vi "NetworkStreamReceiverTemplate.vi"() -> ()   [LabVIEW 2014]
doc: "Use this template to build a producer/consumer design pattern. Use this template when you need to execute a process, such as data analysis, when a data source, such as a triggered acquisition, produces data at an uneven rate and you need to execute the process when the data becomes available."
uses:
  NetworkStreamReceiverState.ctl
  NetworkStreamStateMachineVariable.ctl
  NetworkStreamData.ctl
  NetworkStreamReceiverMainQueueCluster.ctl
  NetworkStreamReceiverStatusEventCluster.ctl
  <vilib>/dex/Stream Element Allocation Mode.ctl
  NetworkStream.lvlib
panel:
  out "Random Session Hash":u64
  out "Network Stream State Indicator":T1
  in  "stop":bool
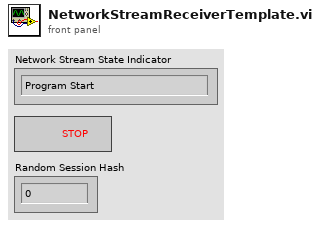
[diagram p1: front panel]
types:
  T1 = typedef "NetworkStream.lvlib/NetworkStreamReceiverState.ctl" = enum16{"Program Start", "Waiting for connection", "Connected", "Connection lost", "Exit", "Unhandled Exception"}
  T2 = typedef "NetworkStream.lvlib/NetworkStreamReceiverStatusEventCluster.ctl" = cluster{"Status":string, "Data":variant, "SequenceNumber":u64}
  T3 = typedef "NetworkStream.lvlib/NetworkStreamReceiverMainQueueCluster.ctl" = cluster{"Command":string, "Data":variant, "SequenceNumber":u64}
  T4 = typedef "NetworkStream.lvlib/NetworkStreamStateMachineVariable.ctl" = cluster{"Network Stream Reader Endpoint":refnum<k21>, "Last Received Sequence Number":u64}
  T5 = typedef "NetworkStream.lvlib/NetworkStreamData.ctl" = cluster{"Command/Status":string, "Data":variant, "Session Hash":u64, "Sequence Number":u64}
  T6 = typedef "Stream Element Allocation Mode.ctl" = u32
  T7 = cluster{"Command/Status":string, "Data":variant, "Sequence Number":u64}
  T8 = cluster{"Status":string, "Data":variant, "Random Session Hash":u64, "SequenceNumberOfFinishedCommand":u64}
  T9 = cluster{"Command":string, "Data":variant, "SequenceNumberOfCommand":u64}
  T10 = cluster{string, "Variant":variant, "SequenceNumber":u64}
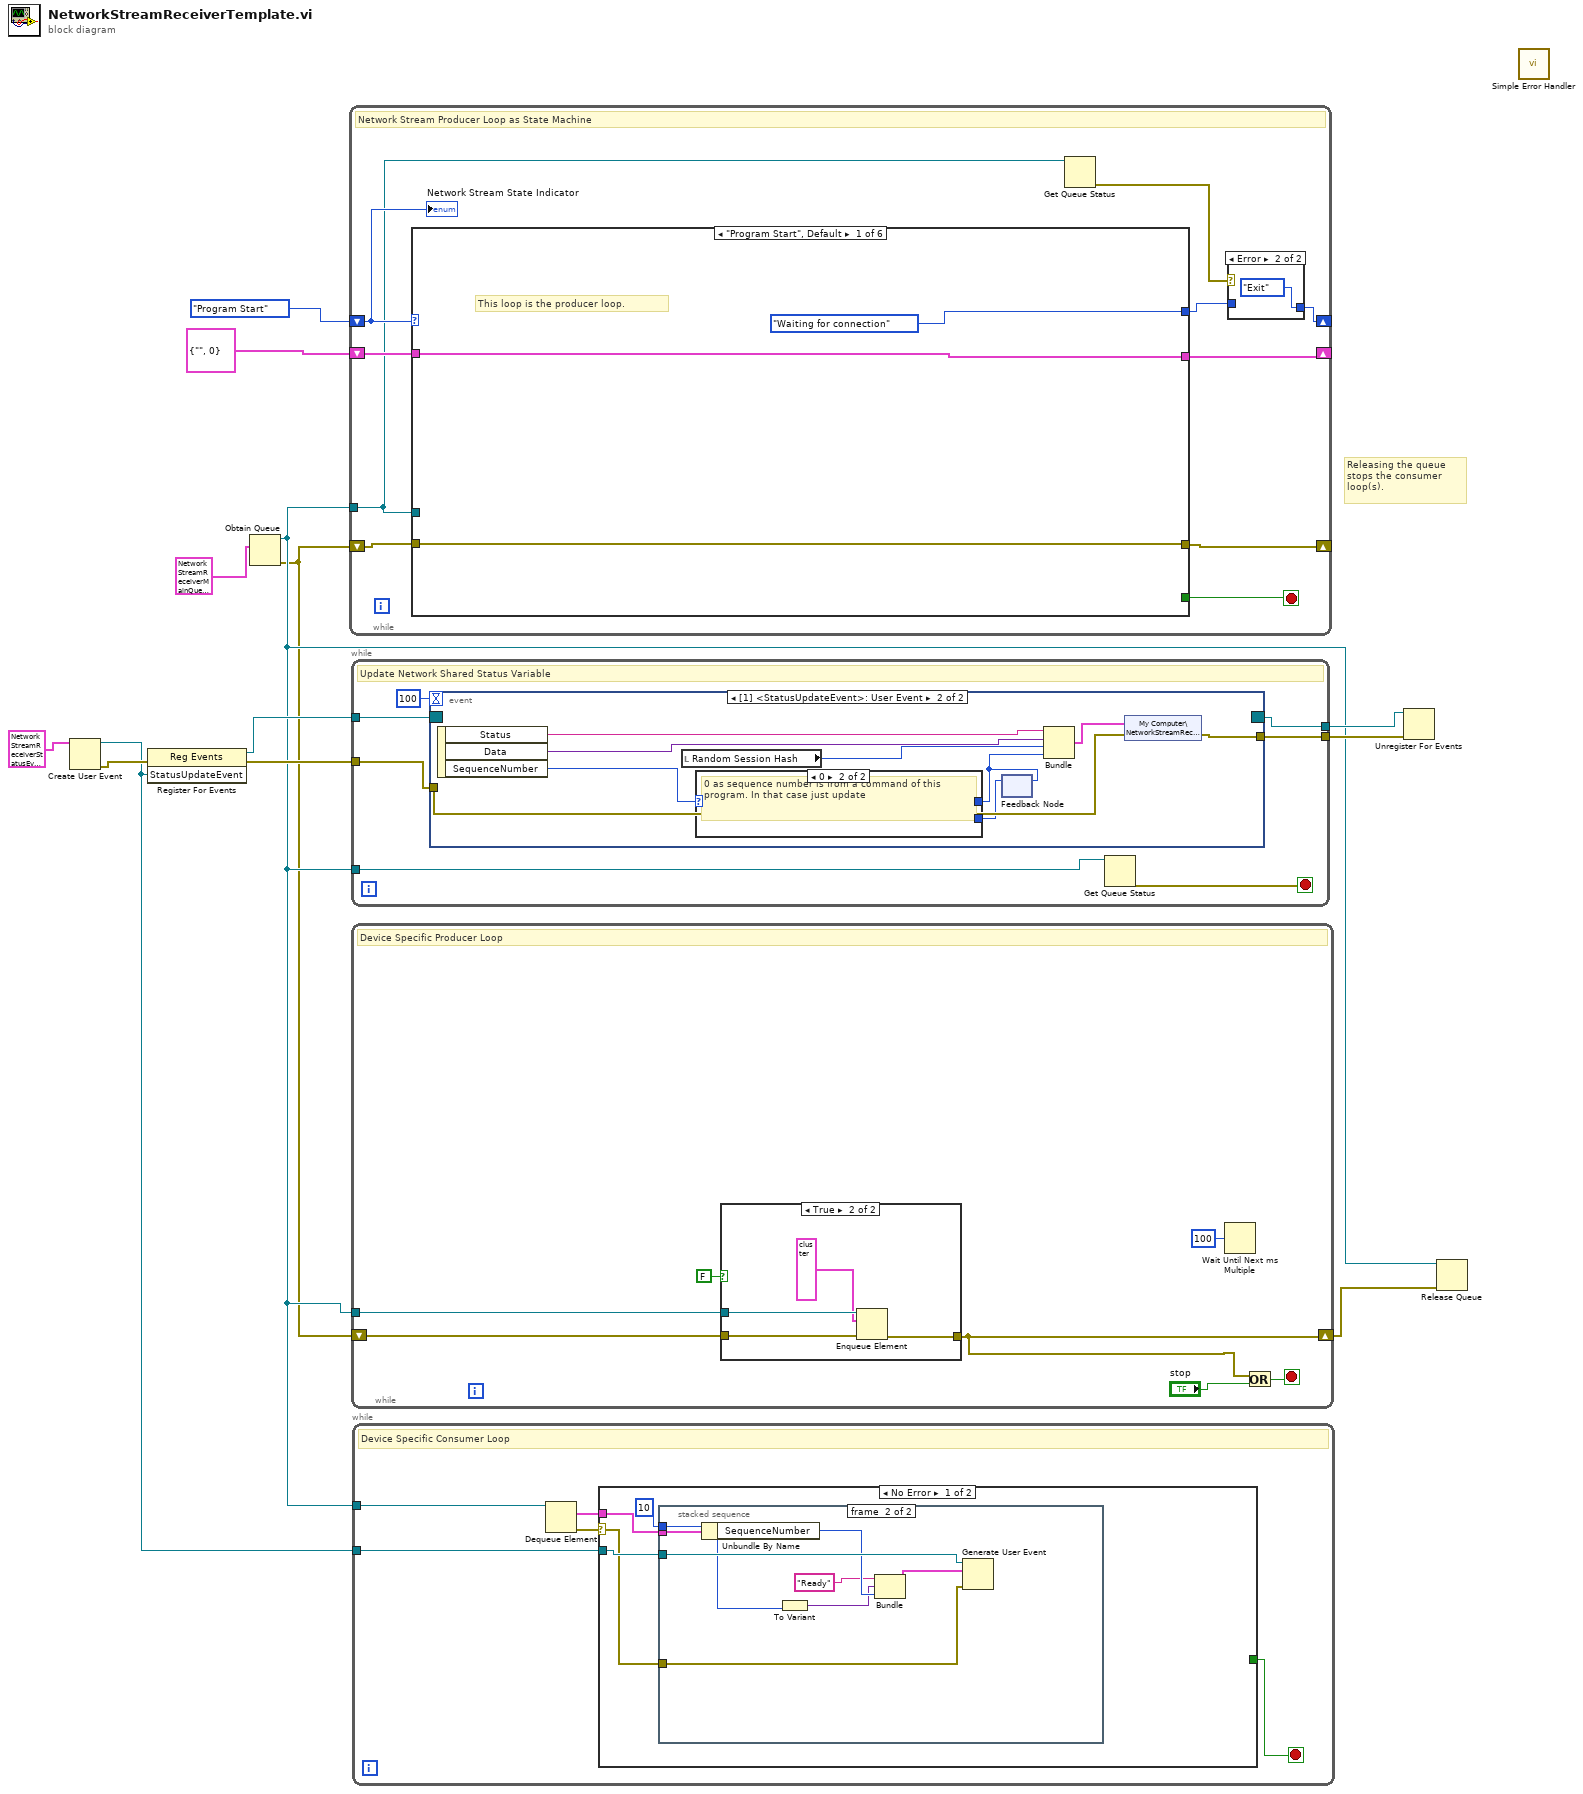
[diagram p0: block diagram]
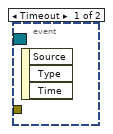
[diagram p3: hidden frame]
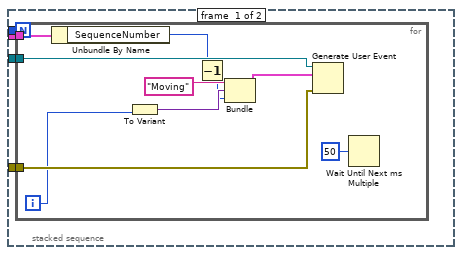
[diagram p5: hidden frame]
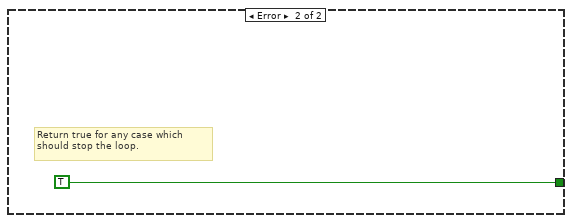
[diagram p6: hidden frame]
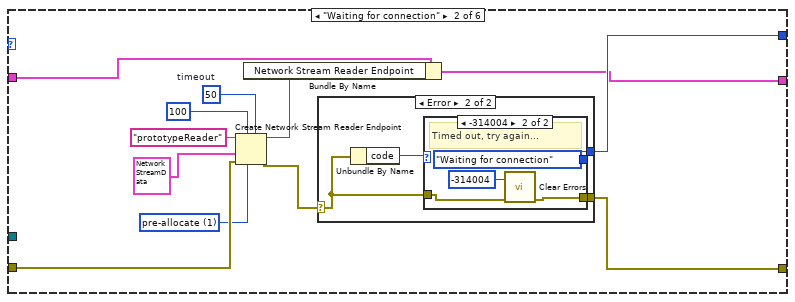
[diagram p8: hidden frame]
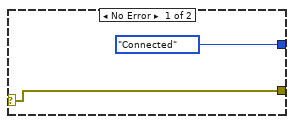
[diagram p9: hidden frame]
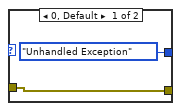
[diagram p10: hidden frame]
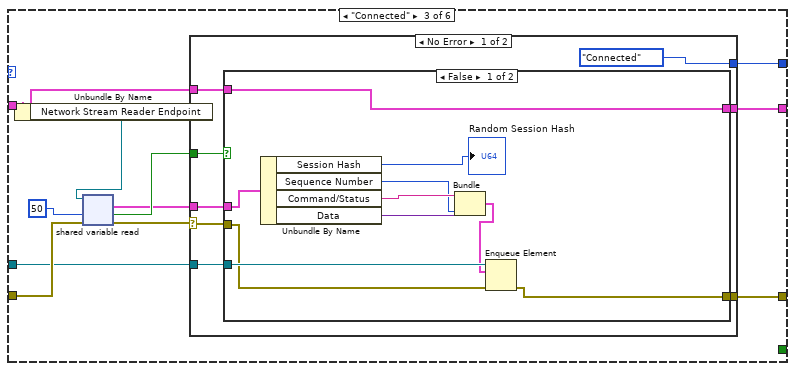
[diagram p11: hidden frame]
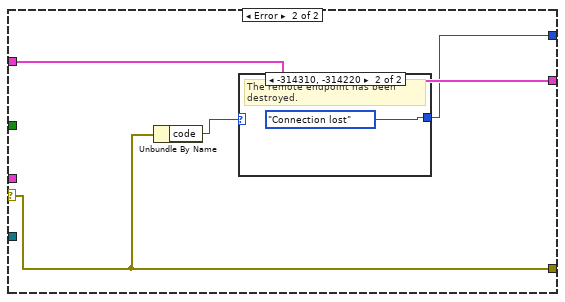
[diagram p13: hidden frame]
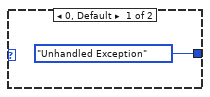
[diagram p14: hidden frame]
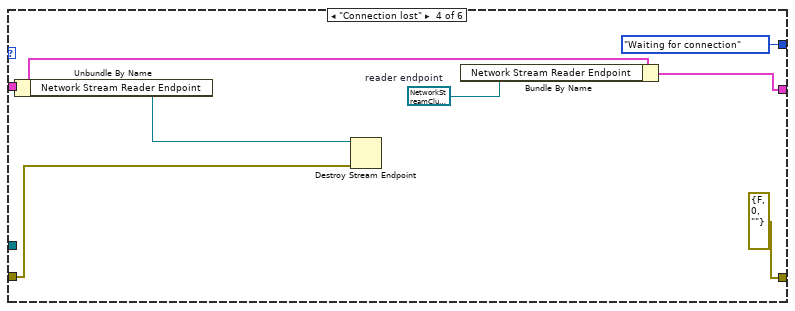
[diagram p15: hidden frame]
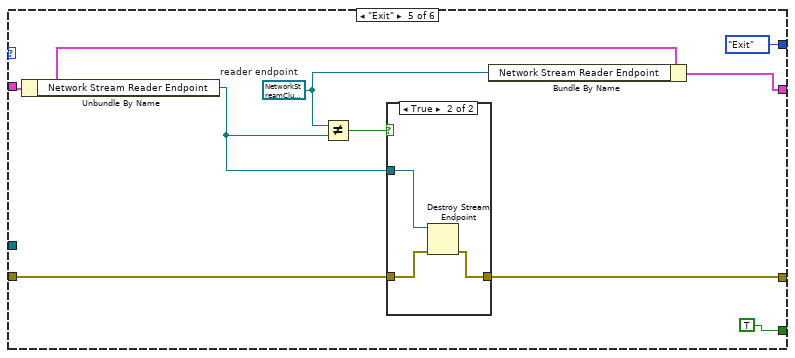
[diagram p16: hidden frame]
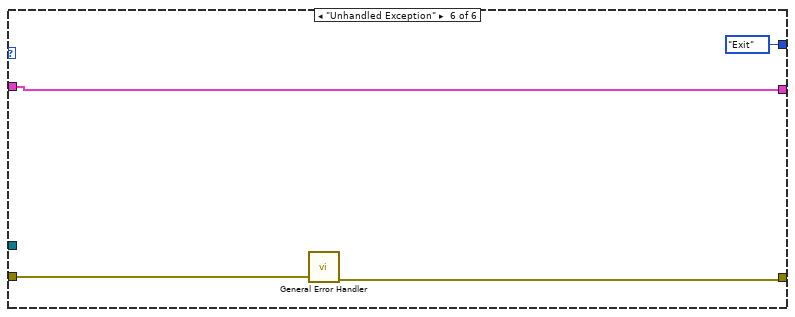
[diagram p18: hidden frame]
diagram:
  # "Releasing the queue stops the consumer loop(s)."
  n1 = Create User Event(user event datatype=T2 {"Status"="", "Data"=variant, "SequenceNumber"=0} ("StatusUpdateEvent")) -> (user event=w1:refnum<user-event>, error out=w10:errorcluster)  [unwired: 1 in]
  n2 = register-events(error in=w10, w1) -> (reference out=w9:refnum<event-registration>, error out=w6:errorcluster)  [unwired: 1 in]
  n3 = Obtain Queue(element data type=T3 {"Command"="", "Data"=variant, "SequenceNumber"=0}) -> (queue out=w4:refnum<queue>, error out=w3:errorcluster)  [unwired: 4 in, 1 out]
  n4 = while {
    shift-right: [w16] -> _
    shift-left: w3 -> [w17]
    shift-right: [w21] -> _
    shift-left: T4 {"Network Stream Reader Endpoint"="", "Last Received Sequence Number"=0} ("StateMachineVariable") -> [w22]
    shift-right: [w19] -> _
    shift-left: NetworkStreamReceiverState."Program Start" -> [w23]
    tunnel: w4 -> [w15]
    stop <- w18 stop-if-true
    # "This loop is the producer loop."
    # "Network Stream Producer Loop as State Machine"
    n5 = case shown="\"Program Start\", Default" w23 {
      tunnel: [NetworkStreamReceiverState."Waiting for connection" w34 w56 NetworkStreamReceiverState."Waiting for connection" NetworkStreamReceiverState."Exit" NetworkStreamReceiverState."Exit"] -> w20
      tunnel: w17 -> [w27 w36 w60 w96 w105 w113]
      tunnel: [w27 w33 w57 errorcluster {"status"=FALSE, "code"=0, "source"=""} ("error out") w104 w112] -> w16
      tunnel: w22 -> [w26 w32 w55 w93 w102 w111]
      tunnel: [w26 w30 w54 w91 w103 w111] -> w21
      tunnel: [_ _ _ _ TRUE _] -> w18
      tunnel: w15 -> [_ _ w53 _ _ _]
      frame "Program Start", Default {
      }
      frame "Waiting for connection" {
        w29 = T6 1 items=["allocate as needed", "pre-allocate"] ("element allocation mode")
        w40 = 50  # timeout
        n6 = Create Network Stream Reader Endpoint(5:w40, 6:w29, 7:100 ("reader buffer size"), 8:w36, 9:T5 {"Command/Status"="", "Data"=variant, "Session Hash"=0, "Sequence Number"=0} ("NetworkStreamCluster"), 11:"prototypeReader" ("reader name")) -> (0:w35:errorcluster, 3:w31:refnum<k21>)  [unwired: 1 in]
        n7 = Bundle By Name(cluster=w32, "Network Stream Reader Endpoint"=w31) -> (w30:T4)
        n8 = case shown="Error" w35 {
          selector: w35 -> [w41 w44]
          tunnel: [NetworkStreamReceiverState."Connected" w46] -> w34
          tunnel: [w41 w43] -> w33
          frame No Error {
          }
          frame Error {
            n9 = Unbundle By Name(w44) -> ("code"=w45:i32)
            n10 = case shown="-314004" w45 {
              tunnel: [NetworkStreamReceiverState."Unhandled Exception" NetworkStreamReceiverState."Waiting for connection"] -> w46
              tunnel: w44 -> [w47 w50]
              tunnel: [w47 w49] -> w43
              frame 0, Default {
              }
              frame -314004 {
                # "Timed out, try again..."
                n11 = call <vilib>:"Clear Errors.vi"("error in (no error)"=w50, "specific error code to clear (0: all)"=-314004) -> ("error out"=w49:errorcluster)  [unwired: 4 in, 1 out]
              }
            }
          }
        }
      }
      frame "Connected" {
        n12 = Unbundle By Name(w55) -> ("Network Stream Reader Endpoint"=w59:refnum<k21>)
        n13 = shared-variable-read(w59, w60, 50 ("timeout ms (-1)")) -> (w58:errorcluster, w62:bool, w61:T5)  [unwired: 1 out]
        n14 = case shown="No Error" w58 {
          selector: w58 -> [w69 w86]
          tunnel: w62 -> [w71 _]
          tunnel: w61 -> [w70 _]
          tunnel: [w68 w86] -> w57
          tunnel: [NetworkStreamReceiverState."Connected" w84] -> w56
          tunnel: w55 -> [w66 w87]
          tunnel: [w65 w87] -> w54
          tunnel: w53 -> [w64 _]
          frame No Error {
            n15 = case shown="False" w71 {
              tunnel: [w78 w83] -> w68
              tunnel: w69 -> [w79 w83]
              tunnel: w70 -> [w81 _]
              tunnel: w66 -> [w72 w82]
              tunnel: [w72 w82] -> w65
              tunnel: w64 -> [w80 _]
              frame False {
                n16 = Unbundle By Name(w81) -> ("Session Hash"=→"Random Session Hash":u64, "Sequence Number"=w74:u64, "Command/Status"=w77:string, "Data"=w76:variant)
                n17 = Bundle("Command/Status"=w77, "Data"=w76, "Sequence Number"=w74) -> (w75:T7)  [unwired: 1 in]
                n18 = Enqueue Element(queue=w80, element=w75, error in (no error)=w79) -> (error out=w78:errorcluster)  [unwired: 1 in, 2 out]
              }
              frame True {
              }
            }
          }
          frame Error {
            n19 = Unbundle By Name(w86) -> ("code"=w85:i32)
            n20 = case shown="-314310, -314220" w85 {
              tunnel: [NetworkStreamReceiverState."Unhandled Exception" NetworkStreamReceiverState."Connection lost"] -> w84
              frame 0, Default {
              }
              frame -314310, -314220 {
                # "The remote endpoint has been destroyed."
              }
            }
          }
        }
      }
      frame "Connection lost" {
        w92 = refnum<k21> refnum  # reader endpoint
        n21 = Unbundle By Name(w93) -> ("Network Stream Reader Endpoint"=w95:refnum<k21>)
        n22 = Destroy Stream Endpoint(8:w96, 11:w95) -> ()  [unwired: 1 out]
        n23 = Bundle By Name(cluster=w93, "Network Stream Reader Endpoint"=w92) -> (w91:T4)
      }
      frame "Exit" {
        w97 = refnum<k21> refnum  # reader endpoint
        n24 = Unbundle By Name(w102) -> ("Network Stream Reader Endpoint"=w100:refnum<k21>)
        n25 = Not Equal?(x=w97, y=w100) -> (x != y?=w99:bool)
        n26 = case shown="True" w99 {
          tunnel: w105 -> [w106 w109]
          tunnel: [w106 w108] -> w104
          tunnel: w100 -> [_ w107]
          frame False {
          }
          frame True {
            n27 = Destroy Stream Endpoint(8:w109, 11:w107) -> (0:w108:errorcluster)
          }
        }
        n28 = Bundle By Name(cluster=w102, "Network Stream Reader Endpoint"=w97) -> (w103:T4)
      }
      frame "Unhandled Exception" {
        n29 = call <vilib>:"General Error Handler.vi"("error in (no error)"=w113) -> ("error out"=w112:errorcluster)  [unwired: 10 in, 4 out]
      }
    }
    n30 = Get Queue Status(queue=w15) -> (error out=w14:errorcluster)  [unwired: 2 in, 7 out]
    n31 = case shown="Error" w14 {
      tunnel: w20 -> [w24 _]
      tunnel: [w24 NetworkStreamReceiverState."Exit"] -> w19
      frame No Error {
      }
      frame Error {
      }
    }
    "Network Stream State Indicator" <- w23
  }
  n32 = while {
    tunnel: w4 -> [w118]
    tunnel: w9 -> [w117]
    tunnel: [w116] -> w8
    tunnel: w6 -> [w115]
    tunnel: [w114] -> w5
    stop <- w119 stop-if-true
    # "Update Network Shared Status Variable"
    n33 = event shown="[1] <StatusUpdateEvent>: User Event" {
      selector: w117 -> [_ _]
      dyn-events: [_ _] -> w116
      timeout: 100 -> [_ _]
      tunnel: w115 -> [_ w129]
      tunnel: [_ w128] -> w114
      event Timeout {
        n34 = event-data() -> ()  [unwired: 1 in, 3 out]
      }
      event User Event {
        n35 = event-data() -> ("Status"=w126:string, "Data"=w124:variant, "SequenceNumber"=w123:u64)  [unwired: 1 in]
        n36 = local read "Random Session Hash"() -> (w125:u64)
        n37 = feedback #1() -> (w121:u64)  [unwired: 1 in]
        n38 = case shown="0" w123 {
          selector: w123 -> [w130 _]
          tunnel: [w130 w131] -> w122
          tunnel: w121 -> [_ w131]
          frame 1, Default {
          }
          frame 0 {
            # "0 as sequence number is from a command of this program. In that case just update"
          }
        }
        n39 = feedback-in #1(w122) -> ()
        n40 = Bundle("Status"=w126, "Data"=w124, "Random Session Hash"=w125, "SequenceNumberOfFinishedCommand"=w122) -> (w127:T8)  [unwired: 1 in]
        n41 = shared-variable "My Computer\\NetworkStreamReceiverTemplate.lvlib\\Status"(w127, error in=w129) -> (error out=w128:errorcluster)
      }
    }
    n42 = Get Queue Status(queue=w118) -> (error out=w119:errorcluster)  [unwired: 2 in, 7 out]
  }
  n43 = while {
    shift-right: [w132] -> w2
    shift-left: w3 -> [w137]
    tunnel: w4 -> [w138]
    stop <- w134 stop-if-true
    # "Device Specific Producer Loop"
    n44 = case shown="True" FALSE {
      tunnel: w138 -> [_ w143]
      tunnel: [w139 w142] -> w132
      tunnel: w137 -> [w139 w140]
      frame False {
      }
      frame True {
        n45 = Enqueue Element(queue=w143, element=T9 {"Command"="", "Data"=variant, "SequenceNumberOfCommand"=0}, error in (no error)=w140) -> (error out=w142:errorcluster)  [unwired: 1 in, 2 out]
      }
    }
    n46 = Wait Until Next ms Multiple(millisecond multiple=u32 100) -> ()  [unwired: 1 out]
    n47 = Or(x=w132, y="stop") -> (x .or. y?=w134:bool)
  }
  n48 = while {
    tunnel: w4 -> [w148]
    tunnel: w1 -> [w144]
    stop <- w145 stop-if-true
    # "Device Specific Consumer Loop"
    n49 = Dequeue Element(queue=w148) -> (element=w146:T3, error out=w147:errorcluster)  [unwired: 2 in, 2 out]
    n50 = case shown="No Error" w147 {
      selector: w147 -> [w151 _]
      tunnel: w146 -> [w150 _]
      tunnel: [_ TRUE] -> w145
      tunnel: w144 -> [w152 _]
      frame No Error {
        n51 = stacked-sequence {
          tunnel: w152 -> [w156 w174]
          tunnel: w151 -> [w155 w173]
          tunnel: w150 -> [w154 w171]
          tunnel: 10 -> [w153 w167]
          frame #0 {
            n52 = for {
              N: w153 -> [_]
              tunnel: w156 -> [w166]
              tunnel: w155 -> [w165]
              tunnel: w154 -> [w163]
              i -> [w158]
              n53 = Unbundle By Name(w163) -> ("SequenceNumber"=w162:u64)
              n54 = To Variant(anything=w158) -> (Variant=w160:variant)
              n55 = Decrement(x=w162) -> (x-1=w159:u64)
              n56 = Bundle("Moving", "Variant"=w160, w159) -> (w164:cluster{string, "Variant":variant, u64})  [unwired: 1 in]
              n57 = Generate User Event(user event=w166, event data cluster=w164, error in=w165) -> ()  [unwired: 1 in, 2 out]
              n58 = Wait Until Next ms Multiple(millisecond multiple=u32 50) -> ()  [unwired: 1 out]
            }
          }
          frame #1 {
            n59 = Unbundle By Name(w171) -> ("SequenceNumber"=w170:u64)
            n60 = To Variant(anything=w167) -> (Variant=w168:variant)
            n61 = Bundle("Ready", "Variant"=w168, "SequenceNumber"=w170) -> (w172:T10)  [unwired: 1 in]
            n62 = Generate User Event(user event=w174, event data cluster=w172, error in=w173) -> ()  [unwired: 1 in, 2 out]
          }
        }
      }
      frame Error {
        # "Return true for any case which should stop the loop."
      }
    }
  }
  n63 = Unregister For Events(event registration refnum=w8, error in=w5) -> ()  [unwired: 1 out]
  n64 = Release Queue(queue=w4, error in (no error)=w2) -> ()  [unwired: 1 in, 3 out]
  n65 = call <vilib>:"Simple Error Handler.vi"() -> ()  [unwired: 5 in, 5 out]
